vi "Generated_Classification.vi"(8 "error in (no error)":errorcluster caption="entrée d'erreur (pas d'erreur)", 11 "make_classification":T2={"n_samples"=100, "n_features"=20, "n_informative"=2, "n_redundant"=2, "n_repeated"=0, "n_classes"=2, "n_clusters_per_class"=2, "weights"=[], "flip_y"=0.01, "class_sep"=1.0, "hypercube"=TRUE, "shift"=[], "scale"=[], "shuffle"=TRUE, "random_state"=-1, "Returns"="X"} {"random_state" min=-1; "n_clusters_per_class" min=1; "n_classes" min=1; "n_features" min=1; "n_samples" min=1}) -> (0 "error out":errorcluster, 3 "Data":T1)   [LabVIEW 2020]
doc: "Generate a random n-class classification problem.\n\nThis initially creates clusters of points normally distributed (std=1) about vertices of an n_informative-dimensional hypercube with sides of length 2*class_sep and assigns an equal number of clusters to each class. It introduces interdependence between these features and adds various types of further noise to the data.\n\nWithout shuffling, X horizontally stacks features in the following order: the primary n_informative features, followed by n_redundant linear combinations of the informative features, followed by n_repeated duplicates, drawn randomly with replacement from the informative and redundant features. The remaining features are filled with random noise. Thus, without shuffling, all useful features are contained in the columns X[:, :n_informative + n_redundant + n_repeated].\n\n\nParameters :\n\n- n_samples : int, optional (default=100)\nThe number of samples.\n\n- n_features : int, optional (default=20)\nThe total number of features. These comprise n_informative informative features, n_redundant redundant features, n_repeated duplicated features and n_features-n_informative-n_redundant-n_repeated useless features drawn at random.\n\n- n_informative : int, optional (default=2)\nThe number of informative features. Each class is composed of a number of gaussian clusters each located around the vertices of a hypercube in a subspace of dimension n_informative. For each cluster, informative features are drawn independently from N(0, 1) and then randomly linearly combined within each cluster in order to add covariance. The clusters are then placed on the vertices of the hypercube.\n\n- n_redundant : int, optional (default=2)\nThe number of redundant features. These features are generated as random linear combinations of the informative features.\n\n- n_repeated : int, optional (default=0)\nThe number of duplicated features, drawn randomly from the informative and the redundant features.\n\n- n_classes : int, optional (default=2)\nThe number of classes (or labels) of the classification problem.\n\n- n_clusters_per_class : int, optional (default=2)\nThe number of clusters per class.\n\n- weights : array-like of shape (n_classes,) or (n_classes - 1,), (default=None)\nThe proportions of samples assigned to each class. If None, then classes are balanced. Note that if len(weights) == n_classes - 1, then the last class weight is automatically inferred. More than n_samples samples may be returned if the sum of weights exceeds 1.\n\n- flip_y : float, optional (default=0.01)\nThe fraction of samples whose class is assigned randomly. Larger values introduce noise in the labels and make the classification task harder. Note that the default setting flip_y > 0 might lead to less than n_classes in y in some cases.\n\n- class_sep : float, optional (default=1.0)\nThe factor multiplying the hypercube size. Larger values spread out the clusters/classes and make the classification task easier.\n\n- hypercube : boolean, optional (default=True)\nIf True, the clusters are put on the vertices of a hypercube. If False, the clusters are put on the vertices of a random polytope.\n\n- shift : float, array of shape [n_features] or None, optional (default=0.0)\nShift features by the specified value. If None, then features are shifted by a random value drawn in [-class_sep, class_sep].\n\n- scale : float, array of shape [n_features] or None, optional (default=1.0)\nMultiply features by the specified value. If None, then features are scaled by a random value drawn in [1, 100]. Note that scaling happens after shifting.\n\n- shuffle : boolean, optional (default=True)\nShuffle the samples and the features.\n\n- random_state : int, RandomState instance, default=None=-1\nDetermines random number generation for dataset creation. Pass an int for reproducible output across multiple function calls. See Glossary.\n\nReturns : \n\n- X : array of shape [n_samples, n_features]\nThe generated samples.\n\n- y : array of shape [n_samples]\nThe integer labels for class membership of each sample."
uses:
  Classification.lvclass
panel:
  out "Classification.lvclass":refnum<class "Classification.lvclass">
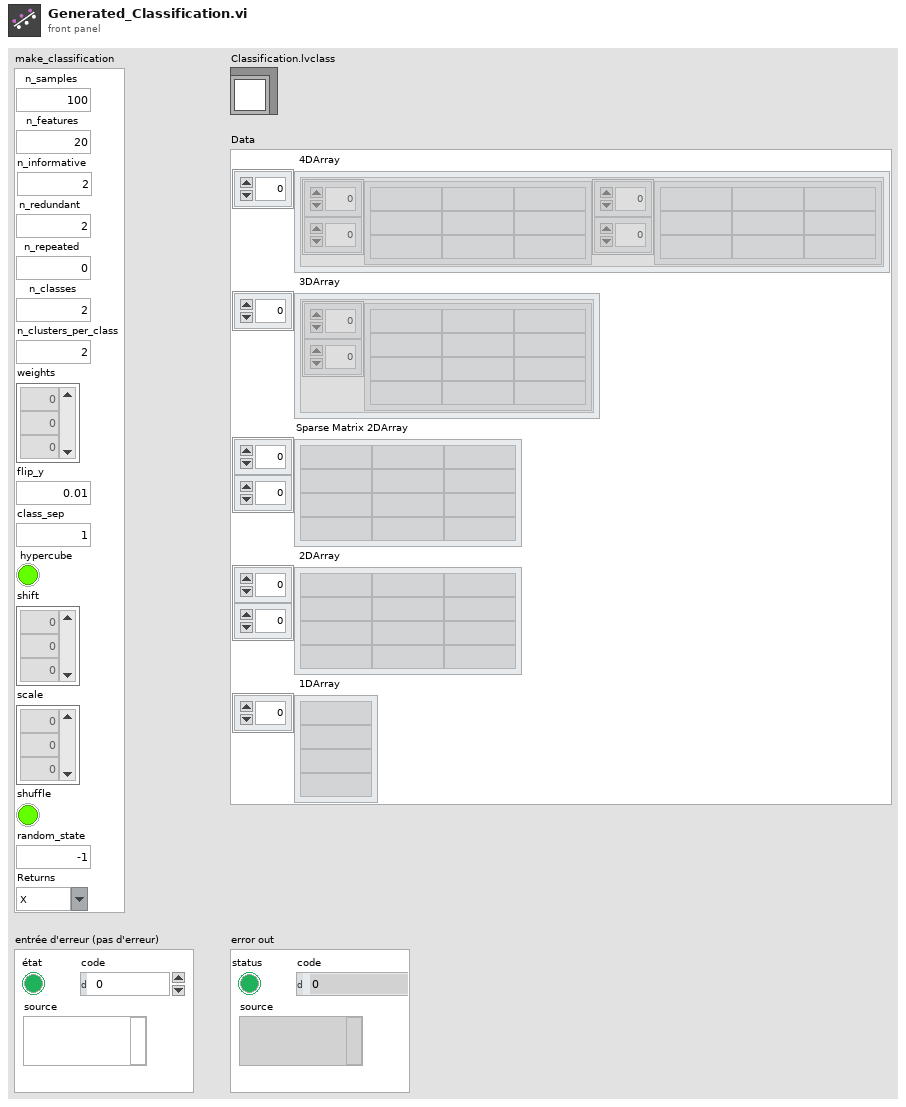
[diagram p1: front panel]
types:
  T1 = cluster{" 4DArray":cluster{"1":string[][], "2":string[][]}[], " 3DArray":cluster{"Tableau":string[][]}[], "Sparse Matrix 2DArray":string[][], " 2DArray":string[][], " 1DArray":string[]}
  T2 = cluster{"n_samples":u32, "n_features":u32, "n_informative":i32, "n_redundant":i32, "n_repeated":i32, "n_classes":u32, "n_clusters_per_class":u32, "weights":i32[], "flip_y":dbl, "class_sep":dbl, "hypercube":bool, "shift":dbl[], "scale":dbl[], "shuffle":bool, "random_state":i32, "Returns":string}
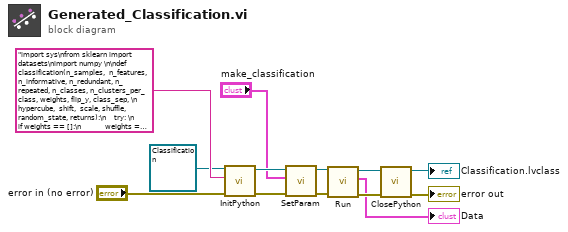
[diagram p0: block diagram]
diagram:
  n1 = call-dynamic "InitPython.vi"("error in (no error)"="error in (no error)", "Python Instruction"="import sys\nfrom sklearn import datasets\nimport numpy \n\ndef classification(n_samples,  n_features, n_informative, n_redundant, n_repeated, n_classes, n_clusters_per_class, weights, flip_y, class_sep, \n          hypercube,  shift,  scale, shuffle, random_state, returns):\n    try: \n        if weights == []:\n            weights = None\n        if random_state == -1:\n            random_state = None\n        if shift == []:\n            shift = None\n        if scale == []:\n            scale = None\n        X, y = datasets.make_classification(n_samples,  n_features, n_informative, n_redundant, n_repeated, n_classes, n_clusters_per_class, weights, flip_y, class_sep, hypercube,  shift,  scale, shuffle, random_state)\n        if returns == 'X':\n            dataX = X.tolist()\n            return str(dataX)\n        else :\n            datay = y.tolist()\n            return str(datay)\n    except:\n        erreur = sys.exc_info()\n        typerr = u\"%s\" % (erreur[0])\n        typerr = typerr[typerr.find(\"'\")+1:typerr.rfind(\"'\")]\n        msgerr = u\"%s\" % (erreur[1])\n        message = str('/!\\\\ {0} : {1}'. format(typerr,msgerr))\n        return message", "Scikit-learn en entrée"=refnum<class "Classification.lvclass"> refnum ("Classification.lvclass")) -> ("error out"=w6:errorcluster, "Scikit-learn en sortie"=w8:refnum<class "Classification.lvclass">)  [unwired: 7 in]
  n2 = call-dynamic "SetParam.vi"("error in (no error)"=w6, "make_classification"="make_classification", "Classification.lvclass"=w8) -> ("error out"=w4:errorcluster, "Classification.lvclass"=w5:refnum<class "Classification.lvclass">)  [unwired: 7 in]
  n3 = call-dynamic "Run.vi"("error in (no error)"=w4, "Classification.lvclass"=w5) -> ("error out"=w10:errorcluster, "Data"=→"Data":T1, "Classification.lvclass"=w9:refnum<class "Classification.lvclass">)  [unwired: 7 in]
  n4 = call-dynamic "ClosePython.vi"("error in (no error)"=w10, "Scikit-learn en entrée"=w9) -> ("error out"=→"error out":errorcluster, "Scikit-learn en sortie"=→"Classification.lvclass":refnum<class "Classification.lvclass">)  [unwired: 8 in]
